vi "Close Statement.vi"(4 "error in (no error)":errorcluster, 7 "Statement Refnum":T1) -> (0 "error out":errorcluster)   [LabVIEW 2011]
doc: "Clotûre la requête et libère le lien associé"
uses:
  SQL Controls/Statement Refnum.ctl
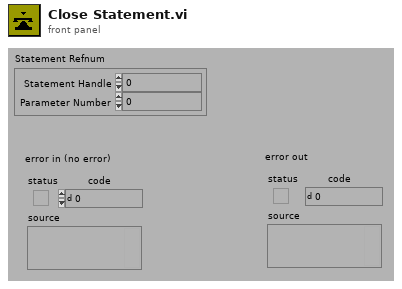
[diagram p1: front panel]
types:
  T1 = typedef "Statement Refnum.ctl" = cluster{"Statement Handle":i32, "Parameter Number":u16}
  T2 = enum16{"NOPE", "SQL_HANDLE_ENV", "SQL_HANDLE_DBC", "SQL_HANDLE_STMT", "SQL_HANDLE_DESC"}
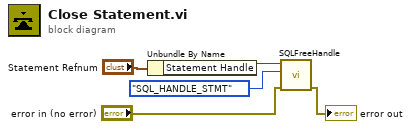
[diagram p0: block diagram]
diagram:
  n1 = Unbundle By Name("Statement Refnum") -> ("Statement Handle"=w3:i32)
  n2 = call "SQLFreeHandle.vi"("error in (no error)"="error in (no error)", "HandleType"=T2."SQL_HANDLE_STMT", "InputHandle"=w3) -> ("error out"=→"error out":errorcluster)  [unwired: 4 out]
